vi "RobotSensorDisplay.vi"() -> ()   [LabVIEW 2018]
uses:
  <vilib>/Rock Robotics/WPI/Ultrasonic/WPI_SonarMB1010AnalogRefNum Registry Get.vi
  <vilib>/Rock Robotics/WPI/Ultrasonic/WPI_SonarMB1010AnalogGetRange.vi
panel:
  out "Pot value":dbl
  out "Right Hab Sensor":dbl
  out "Left Hab Sensor":dbl
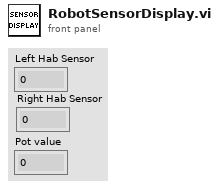
[diagram p1: front panel]
types:
  T1 = typedef "WPI_PotentiometerDevRef.ctl" = cluster{"DevStatus":errorcluster, "Analog Channel":T2, "Invert Output":bool}
  T2 = typedef "FPGA_AIChannel.ctl" = enum8{"AI 0", "AI 1", "AI 2", "AI 3", "AI MXP 0", "AI MXP 1", "AI MXP 2", "AI MXP 3", "Invalid"}
  T3 = typedef "WPI_SonarMB1010AnalogDeviceRef.ctl" = cluster{"AIDeviceRef":T4, "Scaling factor (V/in)":dbl, "Average Bits":u8}
  T4 = typedef "WPI_AnalogChannelDevRef.ctl" = cluster{"DevStatus":errorcluster, "Analog Channel":T2}
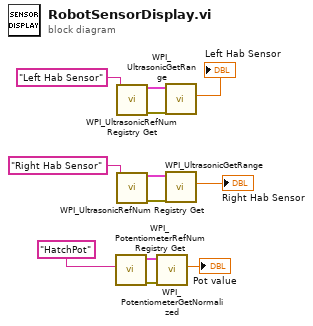
[diagram p0: block diagram]
diagram:
  n1 = call <vilib>:"WPI_PotentiometerRefNum Registry Get.vi"("refnum name"="HatchPot") -> ("error out"=w3:errorcluster, "PotDevRef"=w2:T1)  [unwired: 9 in]
  n2 = call-poly <vilib>:"WPI_UltrasonicRefNum Registry Get.vi"("refnum name"="Left Hab Sensor") -> ("error out"=w12:errorcluster, "SonarMB1010AnalogDevRef"=w11:T3)  [unwired: 9 in]
  n3 = call-poly <vilib>:"WPI_UltrasonicRefNum Registry Get.vi"("refnum name"="Right Hab Sensor") -> ("error out"=w7:errorcluster, "SonarMB1010AnalogDevRef"=w8:T3)  [unwired: 9 in]
  n4 = call <vilib>:"WPI_PotentiometerGetNormalized.vi"("error in"=w3, "PotDevRef"=w2) -> ("Normalized Value"=→"Pot value":dbl)  [unwired: 7 in, 2 out]
  n5 = call-poly <vilib>:"WPI_UltrasonicGetRange.vi"("error in"=w12, "SonarMB1010AnalogDevRef"=w11) -> ("Distance"=→"Left Hab Sensor":dbl)  [unwired: 7 in, 2 out]
  n6 = call-poly <vilib>:"WPI_UltrasonicGetRange.vi"("error in"=w7, "SonarMB1010AnalogDevRef"=w8) -> ("Distance"=→"Right Hab Sensor":dbl)  [unwired: 7 in, 2 out]
